vi "append.vi"(0 "Tree 2":refnum<vi>, 1 "filenames":string[](array[string]), 2 "path":path, 3 "folder names":string[](array[string]), 4 "Open?":bool, 5 "error out":errorcluster) -> (6 "Tree":refnum<vi>, 7 "Array 2":path[](array[path]), 8 "error out 2":errorcluster)   [LabVIEW 2010]
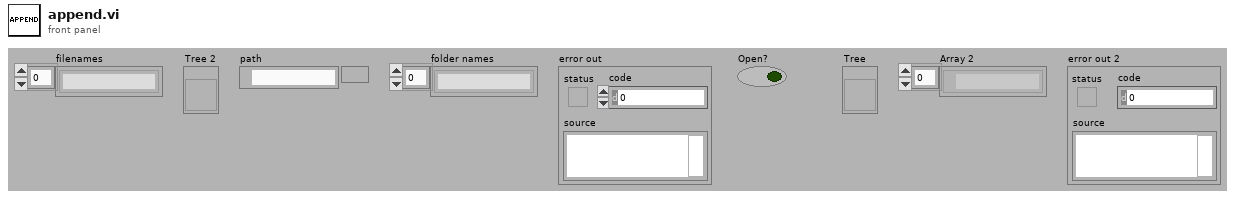
[diagram p1: front panel]
types:
  T1 = cluster{"Left Cell String":string, "Child Text":string[], "Child Tag":string, "Item Indent":i32, "Child Only?":bool, "Glyph Index":i32}[]
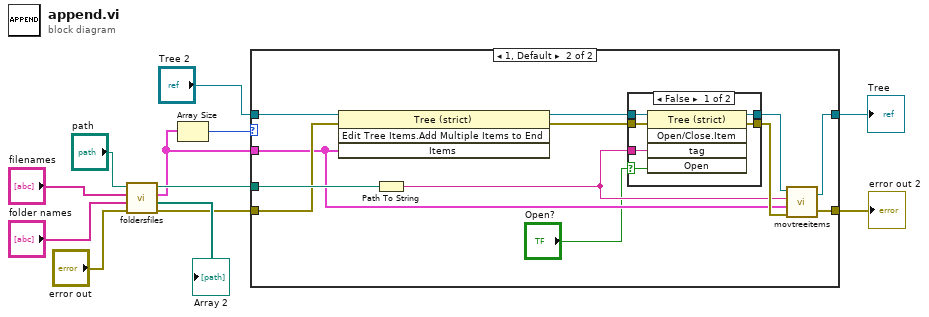
[diagram p0: block diagram]
diagram:
  n1 = call "foldersfiles.vi"("error in"="error out", "folder names"="folder names", "filenames"="filenames", "path"="path") -> ("error out"=w4:errorcluster, "Array 2"=→"Array 2":path[], "Array"=w2:T1, "path out"=w5:path)
  n2 = Array Size(array=w2) -> (size(s)=w1:i32)
  n3 = case shown="1, Default" w1 {
    tunnel: [w13 w26] -> w8
    tunnel: [w14 w23] -> w7
    tunnel: w5 -> [_ w20]
    tunnel: w4 -> [w13 w19]
    tunnel: "Tree 2" -> [w14 w18]
    tunnel: w2 -> [_ w16]
    frame 0 {
    }
    frame 1, Default {
      n4 = invoke on="Invoke Node" class="Tree (strict)" method="Edit Tree Items.Add Multiple Items to End"(reference=w18, error in=w19, "Items"=w16) -> (reference out=w21:refnum<vi>, error out=w24:errorcluster)  [unwired: 1 in, 2 out]
      n5 = Path To String(path=w20) -> (string=w17:string)
      n6 = case shown="False" "Open?" {
        selector: "Open?" -> [w27 _]
        tunnel: [w32 w34] -> w25
        tunnel: w24 -> [w31 w34]
        tunnel: [w30 w33] -> w22
        tunnel: w21 -> [w29 w33]
        tunnel: w17 -> [w28 _]
        frame False {
          n7 = invoke class="Tree (strict)" method="Open/Close.Item"(reference=w29, error in=w31, "tag"=w28, "Open"=w27) -> (reference out=w30:refnum<vi>, error out=w32:errorcluster)  [unwired: 1 in, 3 out]
        }
        frame True {
        }
      }
      n8 = call "movtreeitems.vi"("error out 2"=w25, "Array"=w16, "String"=w17, "Tree 2"=w22) -> ("error out"=w26:errorcluster, "Tree"=w23:refnum<vi>)
    }
  }
  "error out 2" <- w8
  "Tree" <- w7
